vi "Run Tests Programmatically.vi"(4 "Verbose":bool=TRUE, 5 "Silent":bool, 6 "Interactive":bool=TRUE, 7 "Inspect Recursively":bool=TRUE, 9 "Report name":string, 10 "Output Folder":path, 11 "Source Folder":path) -> (0 "error out":errorcluster, 3 "Test Runner":refnum<class "Test Runner.lvclass">)   [LabVIEW 2013, in "Caraya.lvlib"]
uses:
  Caraya.lvlib
  classes/Test Runner/Test Runner.lvclass
  <vilib>/Utility/error.llb/DialogType.ctl
  classes/Test Runner/Test Runner.lvclass/Test Runner.ctl
  classes/Test Runner.Folder/Test Runner.Folder.lvclass
  <userlib>/_OpenG.lib/file/file.llb/File Exists - Scalar__ogtk.vi
  <userlib>/_OpenG.lib/file/file.llb/Valid Path - Traditional__ogtk.vi
  <userlib>/_OpenG.lib/array/array.llb/Delete Elements from 1D Array (Path)__ogtk.vi
  <userlib>/_OpenG.lib/file/file.llb/Strip Path - Arrays__ogtk.vi
  <userlib>/_OpenG.lib/file/file.llb/Strip Path Extension - 1D Array of Strings__ogtk.vi
  <userlib>/_OpenG.lib/file/file.llb/Strip Path Extension - String__ogtk.vi
  <userlib>/_OpenG.lib/file/file.llb/Convert File Extension (String)__ogtk.vi
  classes/Test Report.JUnit/Test Report.JUnit.lvclass
  classes/Test Report.Default/Test Report.Default.lvclass
panel:
  in  "report format":enum16{"Plain text", "JUnit (XML)"}(ring)=enum."JUnit (XML)"
  in  "Defined Tests":i32[](listbox)
  in  "Run Batch Test":bool
  # "CARAYA Batch Testing\n\nFill in the source folder where your tests are and choose the output result options."
  # "Output Configuration"
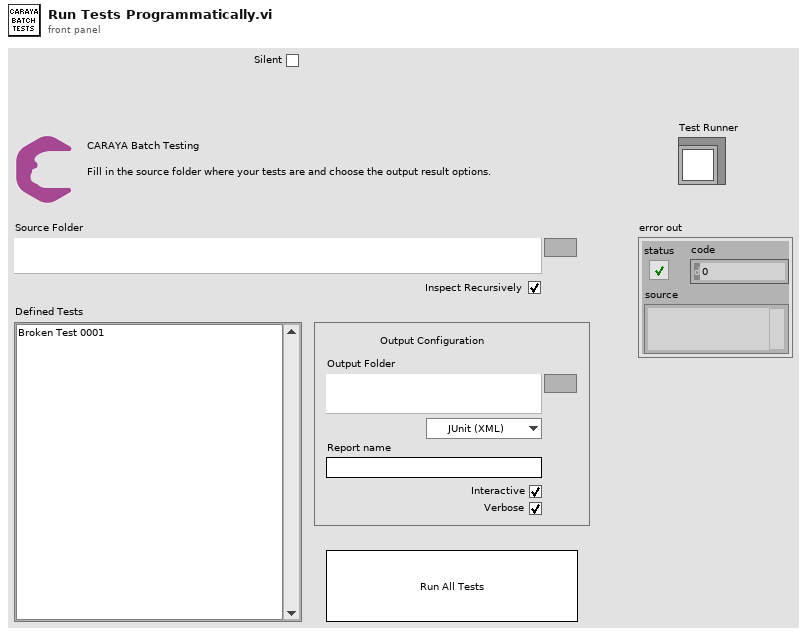
[diagram p1: front panel]
types:
  T1 = enum32{"invalid app kind", "Development System", "Run Time System", "Student Edition", "Embedded LabVIEW", "Evaluation", "Custom"}
  T2 = enum8{"Enabled", "Disabled", "Disabled and Grayed Out"}
  T3 = enum32{"Invalid", "Standard", "Closed", "Hidden", "Minimized", "Maximized"}
  T4 = cluster{"Core":cluster{"Current VI Reference":refnum<vi>, "Close Panel on Exit?":bool}, "Output Folder":path, "Report name":string, "Source Folder":path, "Interactive":bool, "Verbose":bool, "Menu Launch AppRef":refnum<vi>, "Silent":bool, "report format":enum16{"Plain text", "JUnit (XML)"}, "Test Runner":refnum<class "Test Runner.Folder.lvclass">}
  T5 = typedef "DialogType.ctl" = u16
  T6 = cluster{"Current VI Reference":refnum<vi>, "Close Panel on Exit?":bool}
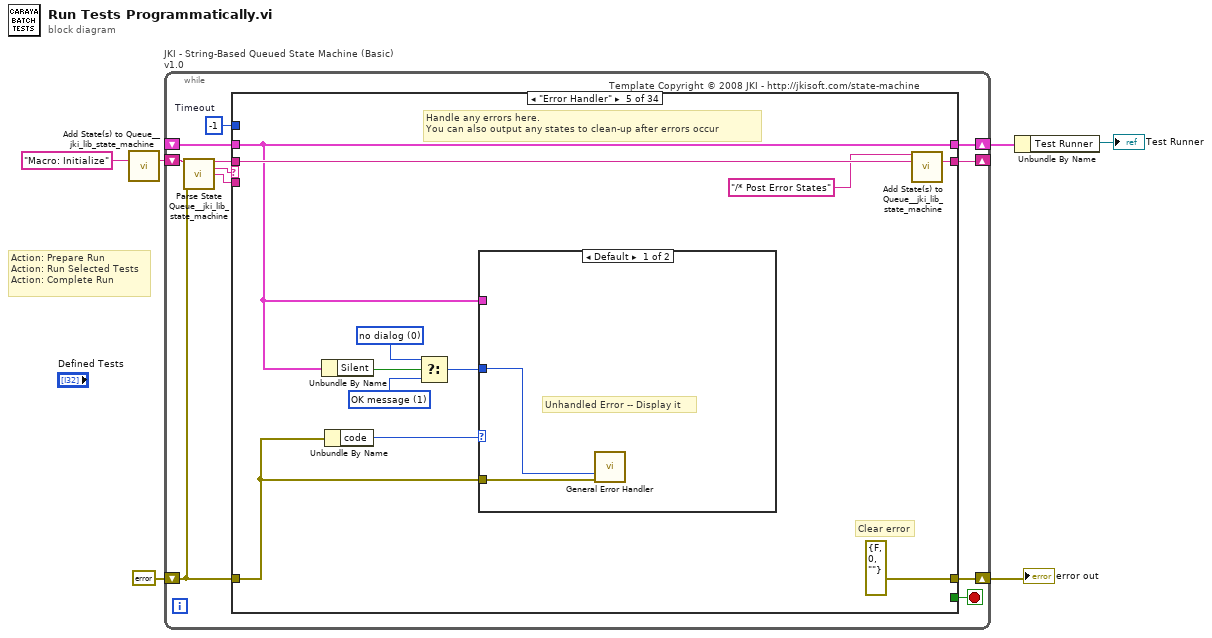
[diagram p0: block diagram]
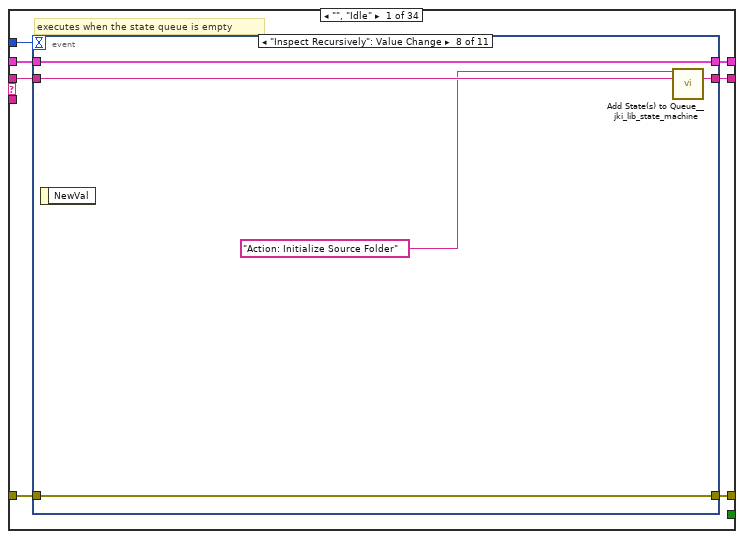
[diagram p2: hidden frame]
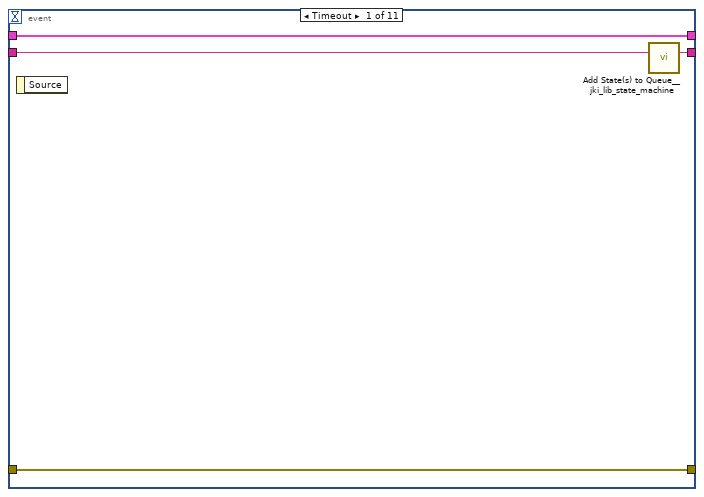
[diagram p3: hidden frame]
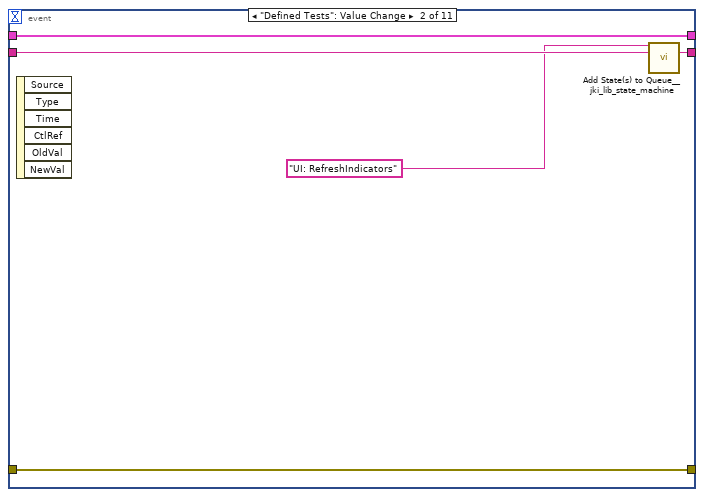
[diagram p4: hidden frame]
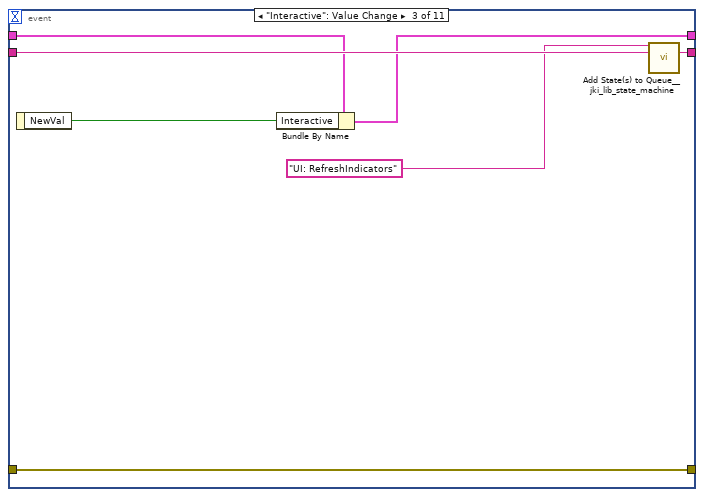
[diagram p5: hidden frame]
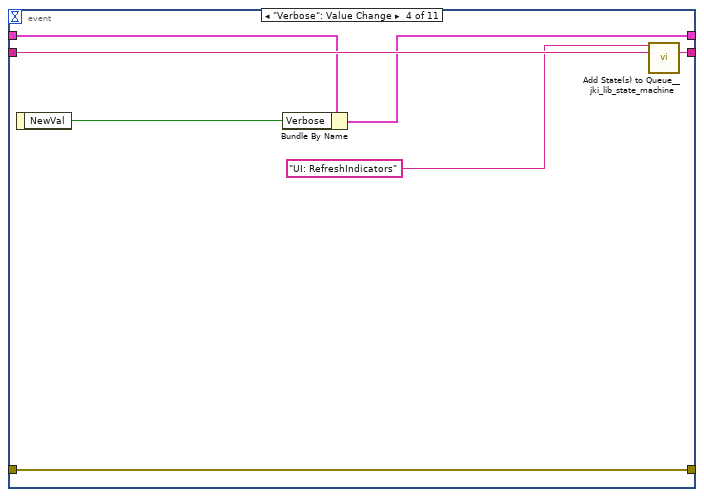
[diagram p6: hidden frame]
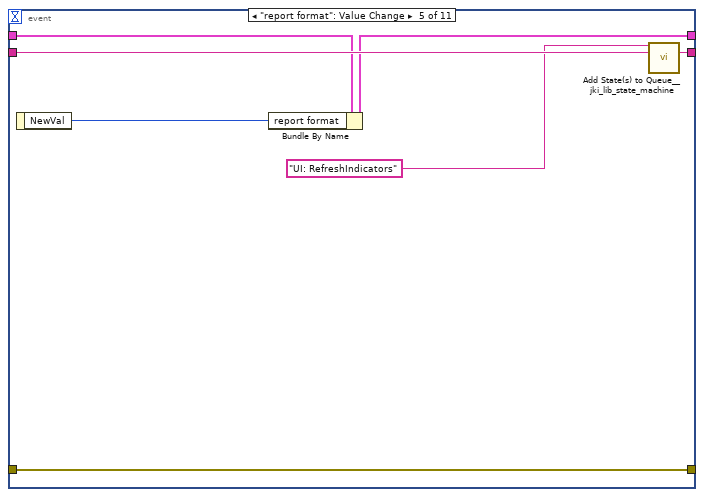
[diagram p7: hidden frame]
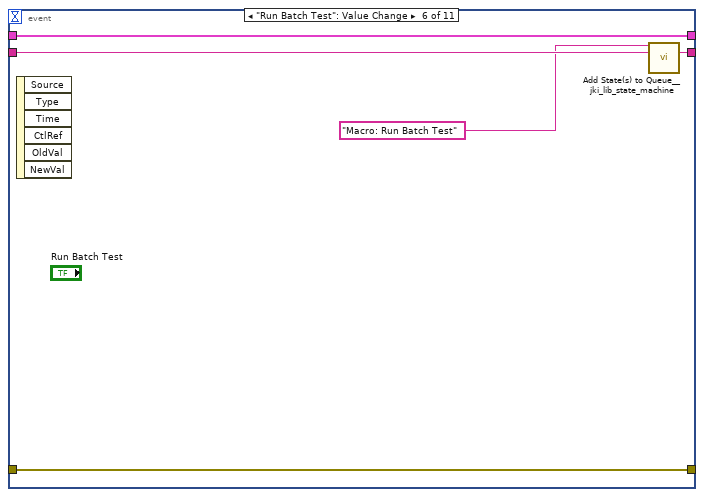
[diagram p8: hidden frame]
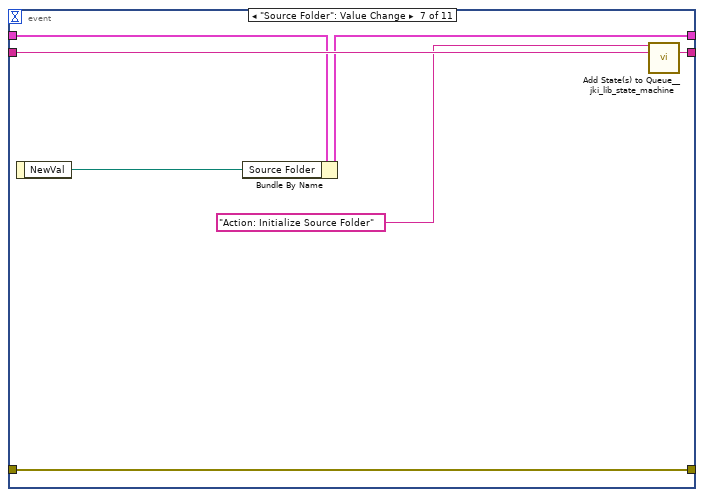
[diagram p9: hidden frame]
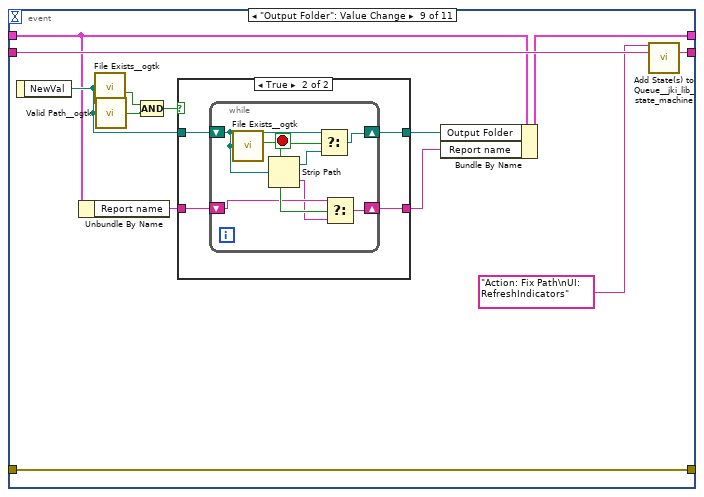
[diagram p10: hidden frame]
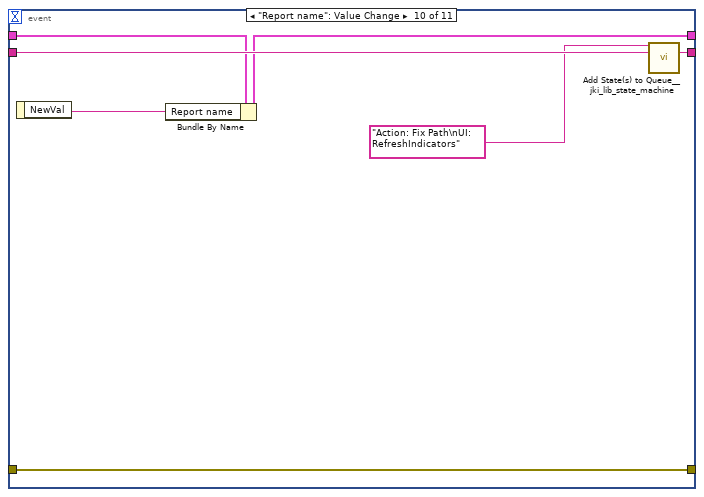
[diagram p12: hidden frame]
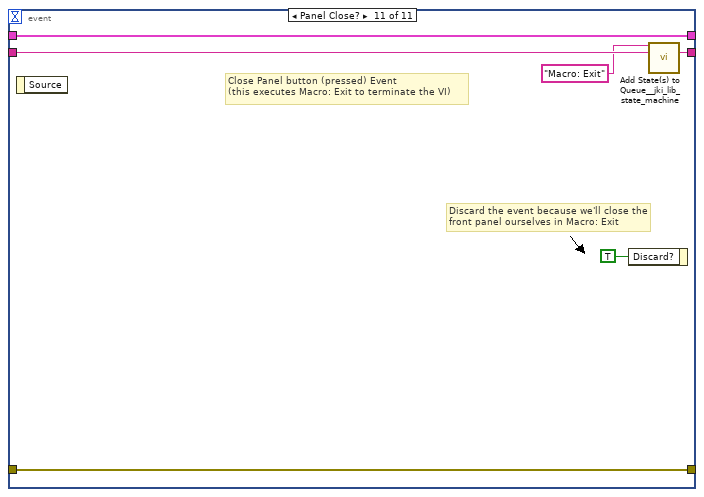
[diagram p13: hidden frame]
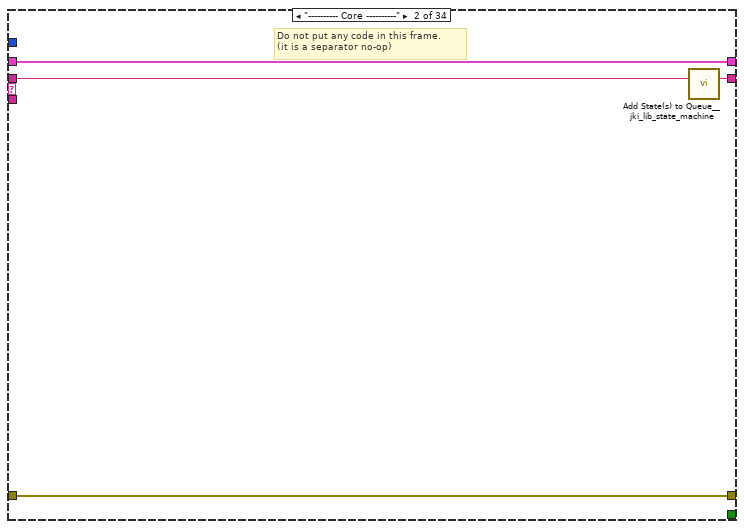
[diagram p14: hidden frame]
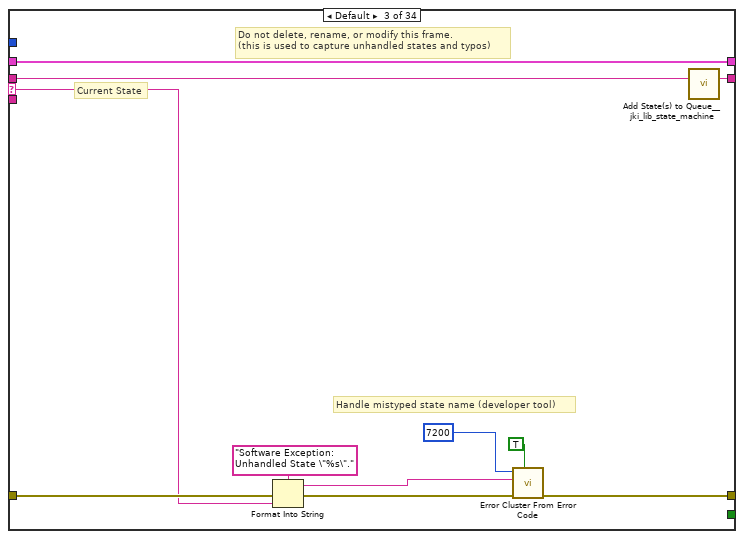
[diagram p15: hidden frame]
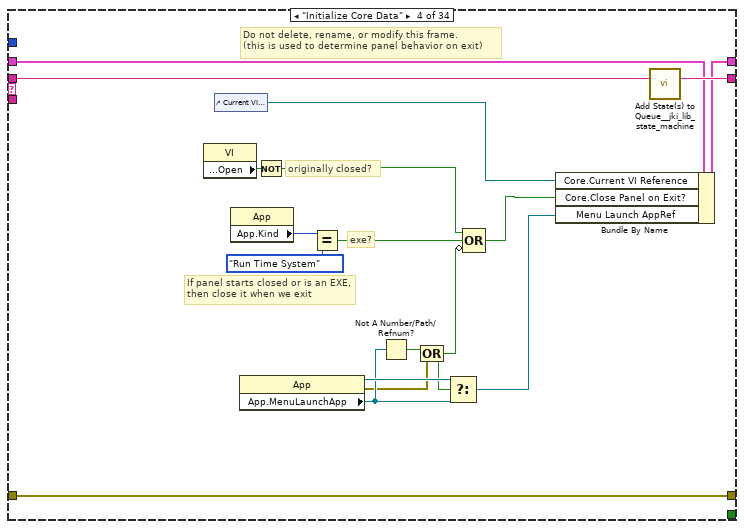
[diagram p16: hidden frame]
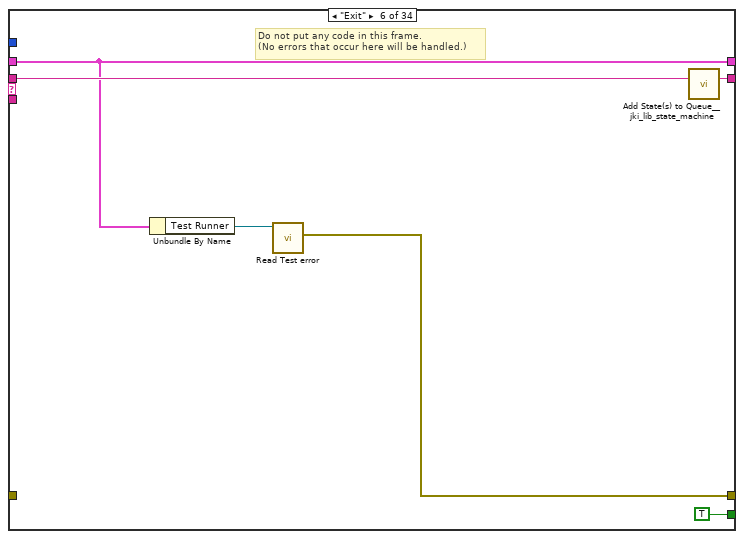
[diagram p18: hidden frame]
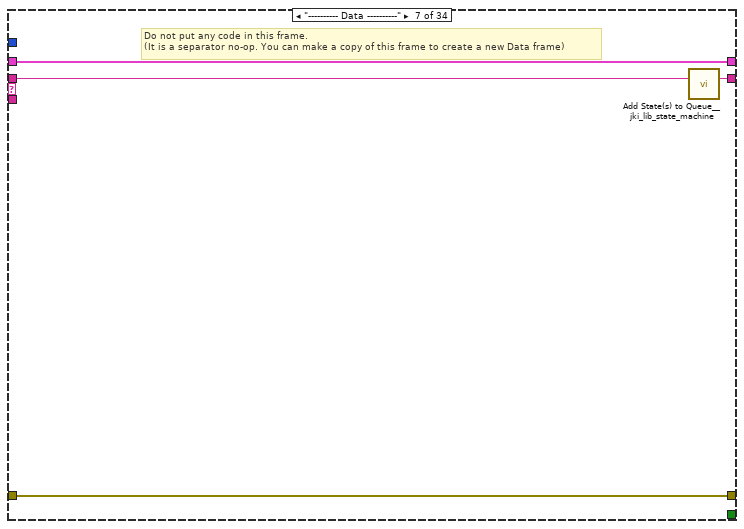
[diagram p19: hidden frame]
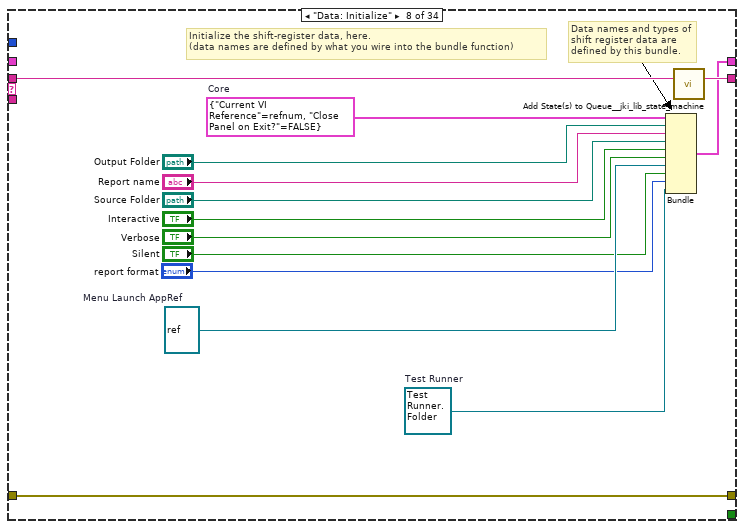
[diagram p20: hidden frame]
diagram:
  # "Action: Prepare Run\nAction: Run Selected Tests\nAction: Complete Run"
  n1 = call <vilib>:"Add State(s) to Queue__jki_lib_state_machine.vi"("State(s) in (\"\")"="Macro: Initialize") -> ("States Out"=w6:string)  [unwired: 14 in]
  n2 = while "JKI - String-Based Queued State Machine (Basic) v1.0" {
    shift-right: [w10] -> w2
    shift-left: _ -> [w9]
    shift-right: [w13] -> w4
    shift-left: errorcluster {"status"=FALSE, "code"=0, "source"=""} ("error IO") -> [w7]
    shift-right: [w12] -> _
    shift-left: w6 -> [w14]
    stop <- w11 stop-if-true
    w8 = -1  # Timeout
    # "Template Copyright © 2008 JKI - http://jkisoft.com/state-machine"
    n3 = call <vilib>:"Parse State Queue__jki_lib_state_machine.vi"("State Queue"=w14, "Error In (no error)"=w7) -> ("Remaining States"=w16:string, "Current State"=w17:string, "Arguments"=w15:string)  [unwired: 11 in]
    n4 = case shown="\"Error Handler\"" w17 {
      selector: w17 -> [_ _ w116 _ _ _ _ _ _ _ _ _ _ _ _ _ _ _ _ _ _ _ _ _ _ _ _ _ _ _ _ _ _ _]
      tunnel: w16 -> [w24 w114 w120 w143 w154 w162 w166 w180 w186 w190 w199 w234 w253 w264 w273 w285 w316 w321 w326 w331 w336 w341 w346 w352 w361 w366 w384 w418 w452 w467 w481 w488 w509 w529]
      tunnel: w15 -> [_ _ _ _ _ _ _ _ _ _ _ _ _ _ w268 w279 _ _ _ _ _ _ _ _ _ _ _ _ _ _ _ _ _ _]
      tunnel: w9 -> [w22 w111 w118 w135 w144 w159 w163 _ w181 w187 w195 w228 w251 w262 w271 w281 w313 w317 w323 w328 w333 w338 w343 w348 w358 w363 w381 w415 w450 w465 w478 w485 w497 w526]
      tunnel: [w21 w112 w122 w140 errorcluster {"status"=FALSE, "code"=0, "source"=""} ("error out") w157 w164 w177 w182 w188 w197 w232 w237 w257 w269 w282 w314 w319 w324 w329 w334 w339 w344 w350 w359 w364 w382 w416 w447 w462 w468 w486 w501 w527] -> w13
      tunnel: w7 -> [w20 w112 w121 w140 w149 _ w164 w177 w183 w188 w197 w232 w237 w258 w270 w283 w314 w319 w324 w329 w334 w339 w344 w350 w359 w364 w382 w416 w443 w460 w469 w486 w502 w527]
      tunnel: [w23 w113 w119 w142 w153 w161 w165 w179 w185 w189 w198 w233 w252 w263 w272 w284 w315 w320 w325 w330 w335 w340 w345 w351 w360 w365 w383 w417 w451 w466 w480 w487 w508 w528] -> w12
      tunnel: [_ _ _ _ _ TRUE _ _ _ _ _ _ _ _ _ _ _ _ _ _ _ _ _ _ _ _ _ _ _ _ _ _ _ _] -> w11
      tunnel: [w19 w111 w118 w141 w144 w159 w163 w178 w181 w187 w194 w227 w250 w262 w271 w281 w313 w317 w323 w328 w333 w338 w343 w348 w358 w363 w375 w414 w449 w464 w477 w485 w503 w526] -> w10
      tunnel: w8 -> [w18 _ _ _ _ _ _ _ _ _ _ _ _ _ _ _ _ _ _ _ _ _ _ _ _ _ _ _ _ _ _ _ _ _]
      frame "", "Idle" {
        # "executes when the state queue is empty"
        n5 = event shown="[7] \"Inspect Recursively\": Value Change" {
          selector: _ -> [_ _ _ _ _ _ _ _ _ _ _]
          dyn-events: _ -> [_ _ _ _ _ _ _ _ _ _ _]
          timeout: w18 -> [_ _ _ _ _ _ _ _ _ _ _]
          tunnel: w24 -> [w28 w33 w40 w47 w54 w59 w66 w71 w84 w104 w110]
          tunnel: [w27 w32 w39 w46 w53 w58 w65 w70 w83 w103 w109] -> w23
          tunnel: w22 -> [w25 w30 w35 w42 w49 w56 w61 w67 w74 w101 w107]
          tunnel: [w26 w31 w38 w45 w52 w57 w64 w69 w82 w102 w108] -> w21
          tunnel: w20 -> [w26 w31 w38 w45 w52 w57 w64 w69 w82 w102 w108]
          tunnel: [w25 w30 w34 w41 w48 w56 w63 w67 w81 w100 w107] -> w19
          event Timeout {
            n6 = event-data() -> ()  [unwired: 1 in, 1 out]
            n7 = call <vilib>:"Add State(s) to Queue__jki_lib_state_machine.vi"("State(s) in (\"\")"=w28) -> ("States Out"=w27:string)  [unwired: 14 in]
          }
          event "Defined Tests": Value Change {
            n8 = event-data() -> ()  [unwired: 1 in, 6 out]
            n9 = call <vilib>:"Add State(s) to Queue__jki_lib_state_machine.vi"("State(s) in Front (\"\")"="UI: RefreshIndicators", "State(s) in (\"\")"=w33) -> ("States Out"=w32:string)  [unwired: 13 in]
          }
          event "Interactive": Value Change {
            n10 = event-data() -> ("NewVal"=w36:bool)  [unwired: 1 in]
            n11 = Bundle By Name(cluster=w35, "Interactive"=w36) -> (w34:T4)
            n12 = call <vilib>:"Add State(s) to Queue__jki_lib_state_machine.vi"("State(s) in Front (\"\")"="UI: RefreshIndicators", "State(s) in (\"\")"=w40) -> ("States Out"=w39:string)  [unwired: 13 in]
          }
          event "Verbose": Value Change {
            n13 = event-data() -> ("NewVal"=w43:bool)  [unwired: 1 in]
            n14 = Bundle By Name(cluster=w42, "Verbose"=w43) -> (w41:T4)
            n15 = call <vilib>:"Add State(s) to Queue__jki_lib_state_machine.vi"("State(s) in Front (\"\")"="UI: RefreshIndicators", "State(s) in (\"\")"=w47) -> ("States Out"=w46:string)  [unwired: 13 in]
          }
          event "report format": Value Change {
            n16 = event-data() -> ("NewVal"=w50:enum16{"Plain text", "JUnit (XML)"})  [unwired: 1 in]
            n17 = Bundle By Name(cluster=w49, "report format"=w50) -> (w48:T4)
            n18 = call <vilib>:"Add State(s) to Queue__jki_lib_state_machine.vi"("State(s) in Front (\"\")"="UI: RefreshIndicators", "State(s) in (\"\")"=w54) -> ("States Out"=w53:string)  [unwired: 13 in]
          }
          event "Run Batch Test": Value Change {
            n19 = event-data() -> ()  [unwired: 1 in, 6 out]
            n20 = call <vilib>:"Add State(s) to Queue__jki_lib_state_machine.vi"("State(s) in Front (\"\")"="Macro: Run Batch Test", "State(s) in (\"\")"=w59) -> ("States Out"=w58:string)  [unwired: 13 in]
          }
          event "Source Folder": Value Change {
            n21 = event-data() -> ("NewVal"=w60:path)  [unwired: 1 in]
            n22 = Bundle By Name(cluster=w61, "Source Folder"=w60) -> (w63:T4)
            n23 = call <vilib>:"Add State(s) to Queue__jki_lib_state_machine.vi"("State(s) in Front (\"\")"="Action: Initialize Source Folder", "State(s) in (\"\")"=w66) -> ("States Out"=w65:string)  [unwired: 13 in]
          }
          event "Inspect Recursively": Value Change {
            n24 = event-data() -> ()  [unwired: 1 in, 1 out]
            n25 = call <vilib>:"Add State(s) to Queue__jki_lib_state_machine.vi"("State(s) in Front (\"\")"="Action: Initialize Source Folder", "State(s) in (\"\")"=w71) -> ("States Out"=w70:string)  [unwired: 13 in]
          }
          event "Output Folder": Value Change {
            n26 = event-data() -> ("NewVal"=w77:path)  [unwired: 1 in]
            n27 = Unbundle By Name(w74) -> ("Report name"=w73:string)
            n28 = call-poly <userlib>:"File Exists__ogtk.vi"("file path"=w77) -> ("exists"=w79:bool)  [unwired: 6 in, 1 out]
            n29 = call-poly <userlib>:"Valid Path__ogtk.vi"("path"=w77) -> ("valid"=w80:bool)
            n30 = Compound Arithmetic op=AND(w79, w80) -> (w78:bool)
            n31 = case shown="True" w78 {
              tunnel: w77 -> [w86 w90]
              tunnel: [w86 w89] -> w76
              tunnel: w73 -> [w85 w88]
              tunnel: [w85 w87] -> w72
              frame False {
              }
              frame True {
                n32 = while {
                  shift-right: [w97] -> w89
                  shift-left: w90 -> [w96]
                  shift-right: [w91] -> w87
                  shift-left: w88 -> [w93]
                  stop <- w94 stop-if-true
                  n33 = call-poly <userlib>:"File Exists__ogtk.vi"("file path"=w96) -> ("is directory"=w94:bool)  [unwired: 6 in, 1 out]
                  n34 = Strip Path(path=w96) -> (stripped path=w95:path, name=w92:string)
                  n35 = Select(t=w96, s=w94, f=w95) -> (s? t:f=w97:path)
                  n36 = Select(t=w93, s=w94, f=w92) -> (s? t:f=w91:string)
                }
              }
            }
            n37 = Bundle By Name(cluster=w74, "Output Folder"=w76, "Report name"=w72) -> (w81:T4)
            n38 = call <vilib>:"Add State(s) to Queue__jki_lib_state_machine.vi"("State(s) in Front (\"\")"="Action: Fix Path\nUI: RefreshIndicators", "State(s) in (\"\")"=w84) -> ("States Out"=w83:string)  [unwired: 13 in]
          }
          event "Report name": Value Change {
            n39 = event-data() -> ("NewVal"=w99:string)  [unwired: 1 in]
            n40 = Bundle By Name(cluster=w101, "Report name"=w99) -> (w100:T4)
            n41 = call <vilib>:"Add State(s) to Queue__jki_lib_state_machine.vi"("State(s) in Front (\"\")"="Action: Fix Path\nUI: RefreshIndicators", "State(s) in (\"\")"=w104) -> ("States Out"=w103:string)  [unwired: 13 in]
          }
          event Panel Close? {
            # "Discard the event because we'll close the front panel ourselves in Macro: Exit"
            # "Close Panel button (pressed) Event\n(this executes Macro: Exit to terminate the VI)"
            n42 = event-data() -> ()  [unwired: 1 in, 1 out]
            n43 = event-data("Discard?"=TRUE) -> ()  [unwired: 1 in, 1 out]
            n44 = call <vilib>:"Add State(s) to Queue__jki_lib_state_machine.vi"("State(s) in Front (\"\")"="Macro: Exit", "State(s) in (\"\")"=w110) -> ("States Out"=w109:string)  [unwired: 13 in]
          }
        }
      }
      frame "---------- Core ----------" {
        # "Do not put any code in this frame.\n(it is a separator no-op)"
        n45 = call <vilib>:"Add State(s) to Queue__jki_lib_state_machine.vi"("State(s) in (\"\")"=w114) -> ("States Out"=w113:string)  [unwired: 14 in]
      }
      frame Default {
        # "Current State"
        # "Do not delete, rename, or modify this frame.\n(this is used to capture unhandled states and typos)"
        # "Handle mistyped state name (developer tool)"
        n46 = Format Into String(format string="Software Exception: Unhandled State \"%s\"." ("message"), error in=w121, w116) -> (resulting string=w124:string, error out=w123:errorcluster)  [unwired: 1 in]
        n47 = call <vilib>:"Error Cluster From Error Code.vi"("show call chain? (False)"=TRUE, "error in (no error)"=w123, "error message (\"\")"=w124, "error code (0)"=7200) -> ("error out"=w122:errorcluster)  [unwired: 5 in]
        n48 = call <vilib>:"Add State(s) to Queue__jki_lib_state_machine.vi"("State(s) in (\"\")"=w120) -> ("States Out"=w119:string)  [unwired: 14 in]
      }
      frame "Initialize Core Data" {
        # "Do not delete, rename, or modify this frame.\n(this is used to determine panel behavior on exit)"
        # "originally closed?"
        # "exe?"
        # "If panel starts closed or is an EXE, then close it when we exit"
        n49 = property class="VI"() -> ("Front Panel.Open"=w139:bool)  [unwired: 2 in, 2 out]
        n50 = control-ref of="Current VI Reference"() -> (w136:refnum<vi>)
        n51 = property class="App"() -> ("App.Kind"=w138:T1)  [unwired: 2 in, 2 out]
        n52 = property class="App"() -> (reference out=w131:refnum<vi>, error out=w128:errorcluster, "App.MenuLaunchApp"=w130:refnum<vi>)  [unwired: 2 in]
        n53 = Not(x=w139) -> (.not. x?=w133:bool)
        n54 = Equal?(x=w138, y=T1."Run Time System" ("Application:Kind")) -> (x = y?=w132:bool)
        n55 = Not A Number/Path/Refnum?(number/path/refnum=w130) -> (NaN/Path/Refnum?=w127:bool)
        n56 = Compound Arithmetic op=OR(w127, w128) -> (w126:bool)
        n57 = Select(t=w131, s=w126, f=w130) -> (s? t:f=w129:refnum<vi>)
        n58 = Compound Arithmetic op=OR(w133, w132, invert w126) -> (w134:bool)
        n59 = Bundle By Name(cluster=w135, "Core.Current VI Reference"=w136, "Core.Close Panel on Exit?"=w134, "Menu Launch AppRef"=w129) -> (w141:T4)
        n60 = call <vilib>:"Add State(s) to Queue__jki_lib_state_machine.vi"("State(s) in (\"\")"=w143) -> ("States Out"=w142:string)  [unwired: 14 in]
      }
      frame "Error Handler" {
        w147 = T5 0 items=["no dialog", "OK message", "continue or stop message", "OK message + warnings", "continue/stop + warnings"] ("type of dialog (OK msg:1)")
        w146 = T5 1 items=["no dialog", "OK message", "continue or stop message", "OK message + warnings", "continue/stop + warnings"] ("type of dialog (OK msg:1)")
        # "Handle any errors here.\nYou can also output any states to clean-up after errors occur"
        # "Clear error"
        n61 = Unbundle By Name(w144) -> ("Silent"=w148:bool)
        n62 = Unbundle By Name(w149) -> ("code"=w150:i32)
        n63 = Select(t=w147, s=w148, f=w146) -> (s? t:f=w145:T5)
        n64 = case shown="Default" w150 {
          tunnel: w149 -> [w156 _]
          tunnel: w145 -> [w155 _]
          tunnel: w144 -> [_ _]
          frame Default {
            # "Unhandled Error -- Display it"
            n65 = call <vilib>:"General Error Handler.vi"("type of dialog (OK msg:1)"=w155, "error in (no error)"=w156) -> ()  [unwired: 9 in, 5 out]
          }
          frame 7000..7999 {
            # "Caraya Error Range"
          }
        }
        n66 = call <vilib>:"Add State(s) to Queue__jki_lib_state_machine.vi"("State(s) in Front (\"\")"="/* Post Error States", "State(s) in (\"\")"=w154) -> ("States Out"=w153:string)  [unwired: 13 in]
      }
      frame "Exit" {
        # "Do not put any code in this frame.\n(No errors that occur here will be handled.)"
        n67 = Unbundle By Name(w159) -> ("Test Runner"=w158:refnum<class "Test Runner.Folder.lvclass">)
        n68 = call "Read Test error.vi"("Test Runner in"=w158) -> ("Test error"=w157:errorcluster)  [unwired: 8 in, 2 out]
        n69 = call <vilib>:"Add State(s) to Queue__jki_lib_state_machine.vi"("State(s) in (\"\")"=w162) -> ("States Out"=w161:string)  [unwired: 14 in]
      }
      frame "---------- Data ----------" {
        # "Do not put any code in this frame.\n(It is a separator no-op. You can make a copy of this frame to create a new Data frame)"
        n70 = call <vilib>:"Add State(s) to Queue__jki_lib_state_machine.vi"("State(s) in (\"\")"=w166) -> ("States Out"=w165:string)  [unwired: 14 in]
      }
      frame "Data: Initialize" {
        w167 = refnum<class "Test Runner.Folder.lvclass"> refnum  # Test Runner
        w175 = refnum<vi> refnum  # Menu Launch AppRef
        w176 = T6 {"Current VI Reference"=refnum, "Close Panel on Exit?"=FALSE}  # Core
        # "Data names and types of shift register data are defined by this bundle."
        # "Initialize the shift-register data, here.\n(data names are defined by what you wire into the bundle function)"
        n71 = Bundle("Core"=w176, "Output Folder"="Output Folder", "Report name"="Report name", "Source Folder"="Source Folder", "Interactive"="Interactive", "Verbose"="Verbose", "Menu Launch AppRef"=w175, "Silent"="Silent", "report format"="report format", "Test Runner"=w167) -> (w178:T4)  [unwired: 1 in]
        n72 = call <vilib>:"Add State(s) to Queue__jki_lib_state_machine.vi"("State(s) in (\"\")"=w180) -> ("States Out"=w179:string)  [unwired: 14 in]
      }
      frame "Data: Cleanup" {
        # "Cleanup any data and references, here.\n(this is called automatically, by the Macro: Exit)"
        n73 = Unbundle By Name(w181) -> ("Core.Current VI Reference"=w184:refnum<vi>)
        n74 = Close Reference(reference=w184, error in (no error)=w183) -> (error out=w182:errorcluster)
        n75 = call <vilib>:"Add State(s) to Queue__jki_lib_state_machine.vi"("State(s) in (\"\")"=w186) -> ("States Out"=w185:string)  [unwired: 14 in]
      }
      frame "---------- UI ----------" {
        # "Do not put any code in this frame.\n(It is a separator no-op. You can make a copy of this frame to create a new UI frame)"
        n76 = call <vilib>:"Add State(s) to Queue__jki_lib_state_machine.vi"("State(s) in (\"\")"=w190) -> ("States Out"=w189:string)  [unwired: 14 in]
      }
      frame "UI: Initialize" {
        # "If Silent, do not set\ninteractive flag to True"
        # "Initialize the User Interface, here.\n(this is called automatically, by the Macro: Init)"
        n77 = Unbundle By Name(w195) -> ("Interactive"=w193:bool, "Silent"=w192:bool)
        n78 = Compound Arithmetic op=AND(w193, invert w192) -> (w191:bool)
        n79 = Bundle By Name(cluster=w195, "Interactive"=w191) -> (w194:T4)
        n80 = call <vilib>:"Add State(s) to Queue__jki_lib_state_machine.vi"("State(s) in Front (\"\")"="UI: Refresh Defined Tests\nAction: Fix Path\nUI: Initialize Path\nUI: RefreshIndicators" ("Text.Text"), "State(s) in (\"\")"=w199) -> ("States Out"=w198:string)  [unwired: 13 in]
      }
      frame "UI: RefreshIndicators" {
        n81 = Unbundle By Name(w228) -> ("Report name"=w210:string, "Output Folder"=w200:path, "Interactive"=w226:bool, "Source Folder"=w205:path, "report format"=w208:enum16{"Plain text", "JUnit (XML)"}, "Test Runner"=w218:refnum<class "Test Runner.Folder.lvclass">)
        n82 = property on="Defined Tests" class="LstBox (strict)"() -> ("Value"=w209:i32[])  [unwired: 2 in, 2 out]
        n83 = local write "Output Folder"(w200) -> ()
        n84 = local write "Report name"(w210) -> ()
        n85 = local write "Source Folder"(w205) -> ()
        n86 = local write "report format"(w208) -> ()
        n87 = call "Read Test VIs.vi"("Test Runner in"=w218) -> ("Test VIs"=w214:path[], "Test Runner out"=w215:refnum<class "Test Runner.Folder.lvclass">)  [unwired: 8 in, 1 out]
        n88 = call-poly <userlib>:"Valid Path__ogtk.vi"("path"=w200) -> ("valid"=w203:bool)
        n89 = call-poly <userlib>:"File Exists__ogtk.vi"("file path"=w200) -> ("is directory"=w202:bool, "exists"=w201:bool)  [unwired: 6 in]
        n90 = Empty Array?(array=w214) -> (empty?=w207:bool)
        n91 = Empty String/Path?(string/path=w200) -> (empty?=w204:bool)
        n92 = Empty Array?(array=w209) -> (empty?=w216:bool)
        n93 = call-poly <userlib>:"Delete Elements from Array__ogtk.vi"("indices"=w209, "array"=w214) -> ("array w/ subset deleted"=w213:path[])  [unwired: 8 in, 1 out]
        n94 = Array Size(array=w209) -> (size(s)=w221:i32)
        n95 = Select(t=path[] [], s=w207, f=w213) -> (s? t:f=w212:path[])
        n96 = Compound Arithmetic op=OR(w207, w204, invert w203, invert w202, invert w201) -> (w206:bool)
        n97 = Format Into String(format string="Run Selected Tests (%d)", w221) -> (resulting string=w219:string)  [unwired: 2 in, 1 out]
        n98 = call "Write Excluded Tests.vi"("Excluded Tests"=w212, "Test Runner in"=w215) -> ("Test Runner out"=w217:refnum<class "Test Runner.Folder.lvclass">)  [unwired: 8 in, 1 out]
        n99 = Select(t="Run All Tests", s=w216, f=w219) -> (s? t:f=w223:string)
        n100 = Bundle By Name(cluster=w228, "Interactive"=w226, "Test Runner"=w217) -> (w227:T4)
        n101 = Select(t="Run Tests", s=w206, f=w223) -> (s? t:f=w224:string)
        n102 = Select(t=T2."Disabled and Grayed Out" ("Disabled"), s=w206, f=T2."Enabled" ("Disabled")) -> (s? t:f=w229:T2)
        n103 = property on="Run Batch Test" class="Bool"("BoolText.Text"=w224) -> ()  [unwired: 2 in, 2 out]
        n104 = property on="Run Batch Test" class="Bool"("DisabledEnum"=w229) -> ()  [unwired: 2 in, 2 out]
        n105 = call <vilib>:"Add State(s) to Queue__jki_lib_state_machine.vi"("State(s) in (\"\")"=w234) -> ("States Out"=w233:string)  [unwired: 14 in]
      }
      frame "UI: Initialize Path" {
        n106 = Unbundle By Name(w251) -> ("Source Folder"=w244:path, "Output Folder"=w238:path)  [unwired: 1 out]
        n107 = call-poly <userlib>:"Valid Path__ogtk.vi"("path"=w238) -> ("valid"=w241:bool)
        n108 = call-poly <userlib>:"File Exists__ogtk.vi"("file path"=w238) -> ("is directory"=w239:bool, "exists"=w240:bool)  [unwired: 6 in]
        n109 = call-poly <userlib>:"Valid Path__ogtk.vi"("path"=w244) -> ("valid"=w247:bool)
        n110 = call-poly <userlib>:"File Exists__ogtk.vi"("file path"=w244) -> ("is directory"=w249:bool, "exists"=w248:bool)  [unwired: 6 in]
        n111 = Compound Arithmetic op=AND(w239, w240, w241) -> (w242:bool)
        n112 = Compound Arithmetic op=AND(w249, w248, w247) -> (w246:bool)
        n113 = Select(t=w238, s=w242, f=path "") -> (s? t:f=w235:path)
        n114 = Select(t=w244, s=w246, f=path "") -> (s? t:f=w243:path)
        n115 = Bundle By Name(cluster=w251, "Source Folder"=w243, "Output Folder"=w235) -> (w250:T4)
        n116 = call <vilib>:"Add State(s) to Queue__jki_lib_state_machine.vi"("State(s) in (\"\")"=w253) -> ("States Out"=w252:string)  [unwired: 14 in]
      }
      frame "UI: Refresh Defined Tests" {
        n117 = Unbundle By Name(w262) -> ("Test Runner"=w260:refnum<class "Test Runner.Folder.lvclass">)
        n118 = call "Read Test VIs.vi"("error in (no error)"=w258, "Test Runner in"=w260) -> ("error out"=w257:errorcluster, "Test VIs"=w259:path[])  [unwired: 7 in, 1 out]
        n119 = call-poly <userlib>:"Strip Path__ogtk.vi"("path"=w259) -> ("name"=w261:string[])  [unwired: 1 out]
        n120 = property on="Defined Tests" class="LstBox (strict)"() -> ("Item Names"=w255:string[])  [unwired: 2 in, 2 out]
        n121 = call-poly <userlib>:"Strip Path Extension__ogtk.vi"("paths"=w261) -> ("roots"=w256:string[])  [unwired: 1 out]
        n122 = Not Equal?(x=w256, y=w255) -> (x != y?=w254:bool)
        n123 = case shown="True" w254 {
          tunnel: w256 -> [_ w267]
          frame False {
          }
          frame True {
            n124 = property on="Defined Tests" class="LstBox (strict)"("Item Names"=w267, "Value"=i32[] [] ("Defined Tests"), "Top Row"=0) -> ()  [unwired: 2 in, 2 out]
          }
        }
        n125 = call <vilib>:"Add State(s) to Queue__jki_lib_state_machine.vi"("State(s) in (\"\")"=w264) -> ("States Out"=w263:string)  [unwired: 14 in]
      }
      frame "UI: Cursor Set" {
        # "Argument"
        # "Set and Unset Cursor Busy.\n(Usage: \"UI: Cursor Set >> Busy|Idle\")"
        n126 = case shown="\"Idle\", Default" w268 {
          tunnel: w270 -> [w275 w277]
          tunnel: [w274 w276] -> w269
          frame "Idle", Default {
            n127 = call <vilib>:"Unset Busy.vi"("error in (no error)"=w275) -> ("error out"=w274:errorcluster)  [unwired: 10 in]
          }
          frame "Busy" {
            n128 = call <vilib>:"Set Busy.vi"("error in (no error)"=w277) -> ("error out"=w276:errorcluster)  [unwired: 9 in, 1 out]
          }
        }
        n129 = call <vilib>:"Add State(s) to Queue__jki_lib_state_machine.vi"("State(s) in (\"\")"=w273) -> ("States Out"=w272:string)  [unwired: 14 in]
      }
      frame "UI: Front Panel State" {
        # "Argument"
        # "Set Front Panel Open or Closed\n(Usage: \"UI: Front Panel State >> Open|Close\")"
        n130 = Unbundle By Name(w281) -> ("Silent"=w278:bool, "Core.Current VI Reference"=w280:refnum<vi>)
        n131 = case shown="\"Open\", Default" w279 {
          tunnel: w283 -> [w287 w307]
          tunnel: [w289 w308] -> w282
          tunnel: w280 -> [w288 w305]
          tunnel: w278 -> [w286 _]
          frame "Open", Default {
            n132 = case shown="False" w286 {
              tunnel: [w295 w302] -> w289
              tunnel: w288 -> [w294 _]
              tunnel: w287 -> [w293 w302]
              frame False {
                n133 = property class="VI"(reference=w294, error in=w293) -> (reference out=w291:refnum<vi>, error out=w292:errorcluster, "Front Panel.Open"=w290:bool)
                n134 = case shown="True" w290 {
                  tunnel: [w298 w301] -> w295
                  tunnel: w292 -> [w297 w301]
                  tunnel: w291 -> [w296 _]
                  frame False {
                    n135 = invoke class="VI" method="FP.Open"(reference=w296, error in=w297, "Activate"=TRUE, "State"=T3."Standard") -> (error out=w298:errorcluster)  [unwired: 1 in, 4 out]
                  }
                  frame True {
                  }
                }
              }
              frame True {
                # "Running Silently. Do not open"
              }
            }
          }
          frame "Close" {
            n136 = property class="VI"(reference=w305, error in=w307) -> (reference out=w304:refnum<vi>, error out=w306:errorcluster, "Front Panel.Open"=w303:bool)
            n137 = case shown="True" w303 {
              tunnel: [w309 w312] -> w308
              tunnel: w306 -> [w309 w311]
              tunnel: w304 -> [_ w310]
              frame False {
              }
              frame True {
                n138 = invoke class="VI" method="FP.Close"(reference=w310, error in=w311) -> (error out=w312:errorcluster)  [unwired: 1 in, 2 out]
              }
            }
          }
        }
        n139 = call <vilib>:"Add State(s) to Queue__jki_lib_state_machine.vi"("State(s) in (\"\")"=w285) -> ("States Out"=w284:string)  [unwired: 14 in]
      }
      frame "---------- Macro ----------" {
        # "Do not put any code in this frame.\n(It is a separator no-op. You can make a copy of this frame to create a new Macro frame)"
        n140 = call <vilib>:"Add State(s) to Queue__jki_lib_state_machine.vi"("State(s) in (\"\")"=w316) -> ("States Out"=w315:string)  [unwired: 14 in]
      }
      frame "Macro: Initialize" {
        w318 = "Data: Initialize\nInitialize Core Data\nUI: Initialize\nUI: Front Panel State >> Open\nAction: Initialize Source Folder\nUI: RefreshIndicators\nMacro: Run Silently?\n"  # Data: Initialize Initialize Core Data UI: Initialize UI: Front Panel State >> Open Action: Initialize Source Folder UI: RefreshIndicators Macro: Run Silently?
        # "Initialization Macro\n(This is called once, when the VI starts)"
        n141 = call <vilib>:"Add State(s) to Queue__jki_lib_state_machine.vi"("State(s) in Front (\"\")"=w318, "State(s) in (\"\")"=w321) -> ("States Out"=w320:string)  [unwired: 13 in]
      }
      frame "Macro: ComputePath" {
        n142 = call <vilib>:"Add State(s) to Queue__jki_lib_state_machine.vi"("State(s) in Front (\"\")"="UI: RefreshIndicators", "State(s) in (\"\")"=w326) -> ("States Out"=w325:string)  [unwired: 13 in]
      }
      frame "Macro: AppendClassName" {
        n143 = call <vilib>:"Add State(s) to Queue__jki_lib_state_machine.vi"("State(s) in Front (\"\")"="UI: RefreshIndicators", "State(s) in (\"\")"=w331) -> ("States Out"=w330:string)  [unwired: 13 in]
      }
      frame "Macro: Find Defined Tests" {
        n144 = call <vilib>:"Add State(s) to Queue__jki_lib_state_machine.vi"("State(s) in Front (\"\")"="Action: Find All Defined Tests\nUI: Refresh Defined Tests\nUI: RefreshIndicators", "State(s) in (\"\")"=w336) -> ("States Out"=w335:string)  [unwired: 13 in]
      }
      frame "Macro: Clear Defined Tests" {
        n145 = call <vilib>:"Add State(s) to Queue__jki_lib_state_machine.vi"("State(s) in Front (\"\")"="Action: Reset\nUI: Refresh Defined Tests\nUI: RefreshIndicators", "State(s) in (\"\")"=w341) -> ("States Out"=w340:string)  [unwired: 13 in]
      }
      frame "Macro: Run Batch Test" {
        n146 = call <vilib>:"Add State(s) to Queue__jki_lib_state_machine.vi"("State(s) in Front (\"\")"="Action: Prepare Run\nAction: Run Selected Tests\nAction: Complete Run", "State(s) in (\"\")"=w346) -> ("States Out"=w345:string)  [unwired: 13 in]
      }
      frame "Macro: Run Silently?" {
        n147 = Unbundle By Name(w348) -> ("Silent"=w347:bool)
        n148 = case shown="True" w347 {
          tunnel: [_ "Macro: Run Batch Test\nMacro: Exit"] -> w349
          frame False {
          }
          frame True {
          }
        }
        n149 = call <vilib>:"Add State(s) to Queue__jki_lib_state_machine.vi"("State(s) in Front (\"\")"=w349, "State(s) in (\"\")"=w352) -> ("States Out"=w351:string)  [unwired: 13 in]
      }
      frame "Macro: Exit" {
        # "Exit Macro\n(This is called once, when the VI exits)"
        n150 = Unbundle By Name(w358) -> ("Core.Close Panel on Exit?"=w354:bool)
        n151 = case shown="True" w354 {
          tunnel: [_ "UI: Front Panel State >> Close"] -> w355
          frame False {
          }
          frame True {
          }
        }
        n152 = call <vilib>:"Add State(s) to Queue__jki_lib_state_machine.vi"("State(s) in Front (\"\")"=w355, "State(s) at Back (\"\")"="Data: Cleanup\nExit") -> ("States Out"=w356:string)  [unwired: 13 in]
        n153 = call <vilib>:"Add State(s) to Queue__jki_lib_state_machine.vi"("State(s) in Front (\"\")"=w356, "State(s) in (\"\")"=w361) -> ("States Out"=w360:string)  [unwired: 13 in]
      }
      frame "---------- Action ----------" {
        n154 = call <vilib>:"Add State(s) to Queue__jki_lib_state_machine.vi"("State(s) in (\"\")"=w366) -> ("States Out"=w365:string)  [unwired: 14 in]
      }
      frame "Action: Fix Path" {
        n155 = Unbundle By Name(w381) -> ("Output Folder"=w377:path, "Report name"=w374:string, "report format"=w372:enum16{"Plain text", "JUnit (XML)"})
        n156 = call-poly <userlib>:"File Exists__ogtk.vi"("file path"=w377) -> ("exists"=w379:bool)  [unwired: 6 in, 1 out]
        n157 = call-poly <userlib>:"Valid Path__ogtk.vi"("path"=w377) -> ("valid"=w380:bool)
        n158 = Compound Arithmetic op=AND(w379, w380) -> (w378:bool)
        n159 = case shown="True" w378 {
          tunnel: w377 -> [w392 w396]
          tunnel: [w392 w395] -> w376
          tunnel: w374 -> [w391 w394]
          tunnel: [w391 w393] -> w368
          frame False {
          }
          frame True {
            n160 = while {
              shift-right: [w403] -> w395
              shift-left: w396 -> [w402]
              shift-right: [w399] -> w393
              shift-left: w394 -> [w400]
              stop <- w398 stop-if-true
              n161 = call-poly <userlib>:"File Exists__ogtk.vi"("file path"=w402) -> ("is directory"=w398:bool)  [unwired: 6 in, 1 out]
              n162 = Strip Path(path=w402) -> (stripped path=w401:path, name=w397:string)
              n163 = Select(t=w400, s=w398, f=w397) -> (s? t:f=w399:string)
              n164 = Select(t=w402, s=w398, f=w401) -> (s? t:f=w403:path)
            }
          }
        }
        n165 = case shown="Default" w368 {
          selector: w368 -> [w404 _]
          tunnel: [w404 w405] -> w369
          frame Default {
          }
          frame "" {
            n166 = Get Date/Time In Seconds() -> (seconds since 1Jan1904=w407:timestamp)
            n167 = Format Into String(format string="%<%Y%m%d_%H%M%S>T", w407) -> (resulting string=w405:string)  [unwired: 2 in, 1 out]
          }
        }
        n168 = call-poly <userlib>:"Strip Path Extension__ogtk.vi"("path"=w368) -> ("root"=w370:string, "extension"=w373:string)
        n169 = case shown="Default" w373 {
          tunnel: w372 -> [_ _ w390]
          tunnel: [enum16{"Plain text", "XML"}."XML" ("report format") enum16{"Plain text", "XML"}."Plain text" ("report format") w390] -> w371
          tunnel: w370 -> [w385 w387 _]
          tunnel: w369 -> [_ _ w389]
          tunnel: [w385 w387 w389] -> w367
          frame "xml" {
          }
          frame "txt" {
          }
          frame Default {
          }
        }
        n170 = Bundle By Name(cluster=w381, "Output Folder"=w376, "Report name"=w367, "report format"=w371) -> (w375:T4)
        n171 = call <vilib>:"Add State(s) to Queue__jki_lib_state_machine.vi"("State(s) in (\"\")"=w384) -> ("States Out"=w383:string)  [unwired: 14 in]
      }
      frame "Action: Initialize Source Folder" {
        n172 = Unbundle By Name(w415) -> ("Source Folder"=w410:path)
        n173 = for {
          N: 2 -> [_]
          tunnel: [w420] -> w411
          shift-right: [w421] -> w409
          shift-left: w410 -> [w422]
          stop <- w420 stop-if-true
          n174 = call-poly <userlib>:"Valid Path__ogtk.vi"("path"=w422) -> ("valid"=w423:bool)
          n175 = call-poly <userlib>:"File Exists__ogtk.vi"("file path"=w422) -> ("exists"=w419:bool)  [unwired: 6 in, 1 out]
          n176 = Compound Arithmetic op=AND(w419, w423) -> (w420:bool)
          n177 = case shown="False" w420 {
            tunnel: w422 -> [_ w428]
            tunnel: [w426 w428] -> w421
            tunnel: [w425 _] -> _
            frame False {
              n178 = property class="App"() -> (error out=w424:errorcluster, "Project.ActiveProject"=w427:refnum<vi>)  [unwired: 2 in, 1 out]
              n179 = property class="Project"(reference=w427, error in=w424) -> (error out=w425:errorcluster, "Path"=w426:path)  [unwired: 1 out]
            }
            frame True {
            }
          }
        }
        n180 = case shown="True" w411 {
          tunnel: w409 -> [w430 w433]
          tunnel: [w430 w432] -> w413
          tunnel: ["Macro: Clear Defined Tests" "Macro: Find Defined Tests"] -> w412
          frame False {
          }
          frame True {
            n181 = while {
              shift-right: [w436] -> w432
              shift-left: w433 -> [w435]
              stop <- w437 stop-if-true
              n182 = call-poly <userlib>:"File Exists__ogtk.vi"("file path"=w435) -> ("is directory"=w437:bool)  [unwired: 6 in, 1 out]
              n183 = Strip Path(path=w435) -> (stripped path=w434:path)  [unwired: 1 out]
              n184 = Select(t=w435, s=w437, f=w434) -> (s? t:f=w436:path)
            }
          }
        }
        n185 = Bundle By Name(cluster=w415, "Source Folder"=w413) -> (w414:T4)
        n186 = call <vilib>:"Add State(s) to Queue__jki_lib_state_machine.vi"("State(s) in Front (\"\")"=w412, "State(s) in (\"\")"=w418) -> ("States Out"=w417:string)  [unwired: 13 in]
      }
      frame "Action: Find All Defined Tests" {
        n187 = Unbundle By Name(w450) -> ("Menu Launch AppRef"=w438:refnum<vi>, "Test Runner"=w446:refnum<class "Test Runner.Folder.lvclass">, "Source Folder"=w444:path)
        n188 = call "Setup TestRunner Folder.vi"("Inspect Recursively (T)"="Inspect Recursively", "error in (no error)"=w443, "Directory to search"=w444, "Test Runner.Folder"=w446) -> ("error out"=w440:errorcluster, "Test Runner.Folder out"=w442:refnum<class "Test Runner.Folder.lvclass">)  [unwired: 6 in]
        n189 = call "Write ApplicationRef.vi"("error in (no error)"=w440, "Application"=w438, "Test Runner in"=w442) -> ("error out"=w439:errorcluster, "Test Runner out"=w441:refnum<class "Test Runner.Folder.lvclass">)  [unwired: 7 in]
        n190 = call "Discover Tests.vi"("error in (no error)"=w439, "Test Runner in"=w441) -> ("error out"=w447:errorcluster, "Test Runner out"=w448:refnum<class "Test Runner.Folder.lvclass">)  [unwired: 8 in]
        n191 = Bundle By Name(cluster=w450, "Test Runner"=w448) -> (w449:T4)
        n192 = call <vilib>:"Add State(s) to Queue__jki_lib_state_machine.vi"("State(s) in (\"\")"=w452) -> ("States Out"=w451:string)  [unwired: 14 in]
      }
      frame "Action: Reset" {
        n193 = Unbundle By Name(w465) -> ("Menu Launch AppRef"=w453:refnum<vi>, "Test Runner"=w459:refnum<class "Test Runner.Folder.lvclass">, "Source Folder"=w461:path)
        n194 = local read "Inspect Recursively"() -> (w458:bool)
        n195 = call "Setup TestRunner Folder.vi"("Inspect Recursively (T)"=w458, "error in (no error)"=w460, "Directory to search"=w461, "Test Runner.Folder"=w459) -> ("error out"=w455:errorcluster, "Test Runner.Folder out"=w457:refnum<class "Test Runner.Folder.lvclass">)  [unwired: 6 in]
        n196 = call "Write ApplicationRef.vi"("error in (no error)"=w455, "Application"=w453, "Test Runner in"=w457) -> ("error out"=w454:errorcluster, "Test Runner out"=w456:refnum<class "Test Runner.Folder.lvclass">)  [unwired: 7 in]
        n197 = call "Discover Tests.vi"("error in (no error)"=w454, "Test Runner in"=w456) -> ("error out"=w462:errorcluster, "Test Runner out"=w463:refnum<class "Test Runner.Folder.lvclass">)  [unwired: 8 in]
        n198 = Bundle By Name(cluster=w465, "Test Runner"=w463) -> (w464:T4)
        n199 = call <vilib>:"Add State(s) to Queue__jki_lib_state_machine.vi"("State(s) in (\"\")"=w467) -> ("States Out"=w466:string)  [unwired: 14 in]
      }
      frame "Action: Run Selected Tests" {
        n200 = Unbundle By Name(w478) -> ("Test Runner"=w479:refnum<class "Test Runner.Folder.lvclass">)
        n201 = property on="Defined Tests" class="LstBox (strict)"() -> ("Value"=w473:i32[])  [unwired: 2 in, 2 out]
        n202 = call "Read Test VIs.vi"("Test Runner in"=w479) -> ("Test VIs"=w475:path[], "Test Runner out"=w476:refnum<class "Test Runner.Folder.lvclass">)  [unwired: 8 in, 1 out]
        n203 = Empty Array?(array=w473) -> (empty?=w472:bool)
        n204 = case shown="False" w472 {
          tunnel: w475 -> [w484 _]
          tunnel: [w483 _] -> w474
          tunnel: w473 -> [w482 _]
          frame False {
            n205 = call-poly <userlib>:"Delete Elements from Array__ogtk.vi"("indices"=w482, "array"=w484) -> ("array w/ subset deleted"=w483:path[])  [unwired: 8 in, 1 out]
          }
          frame True {
          }
        }
        n206 = call "Write Excluded Tests.vi"("Excluded Tests"=w474, "Test Runner in"=w476) -> ("Test Runner out"=w471:refnum<class "Test Runner.Folder.lvclass">)  [unwired: 8 in, 1 out]
        n207 = call "Run.vi"("error in (no error)"=w469, "Test Runner in"=w471) -> ("error out"=w468:errorcluster, "Test Runner out"=w470:refnum<class "Test Runner.Folder.lvclass">)  [unwired: 7 in, 1 out]
        n208 = Bundle By Name(cluster=w478, "Test Runner"=w470) -> (w477:T4)
        n209 = call <vilib>:"Add State(s) to Queue__jki_lib_state_machine.vi"("State(s) in (\"\")"=w481) -> ("States Out"=w480:string)  [unwired: 14 in]
      }
      frame "Action: Complete Run" {
        n210 = call <vilib>:"Add State(s) to Queue__jki_lib_state_machine.vi"("State(s) in (\"\")"=w488) -> ("States Out"=w487:string)  [unwired: 14 in]
      }
      frame "Action: Prepare Run" {
        n211 = Unbundle By Name(w497) -> ("Output Folder"=w504:path, "Report name"=w505:string, "report format"=w507:enum16{"Plain text", "JUnit (XML)"}, "Verbose"=w506:bool)  [unwired: 1 out]
        n212 = Unbundle By Name(w497) -> ("Menu Launch AppRef"=w489:refnum<vi>, "Interactive"=w495:bool, "Test Runner"=w498:refnum<class "Test Runner.Folder.lvclass">, "Source Folder"=w496:path)
        n213 = case shown="\"Plain text\", Default" w507 {
          tunnel: [w512 w519] -> w499
          tunnel: w506 -> [w510 w518]
          tunnel: w505 -> [w514 w525]
          tunnel: w504 -> [w515 w522]
          tunnel: [w511 w521] -> w500
          frame "Plain text", Default {
            n214 = call-poly <userlib>:"Convert File Extension__ogtk.vi"("new ending (none)"="txt", "file name"=w514) -> ("new filename"=w516:string)  [unwired: 1 out]
            n215 = Build Path(base path=w515, name or relative path=w516) -> (appended path=w513:path)
            n216 = call "Create DefaultReport.vi"("Verbose"=w510, "Report Path"=w513) -> ("error out"=w512:errorcluster, "Test Report.Default out"=w511:refnum<class "Test Report.Default.lvclass">)  [unwired: 8 in]
          }
          frame "JUnit (XML)" {
            n217 = call-poly <userlib>:"Convert File Extension__ogtk.vi"("new ending (none)"="xml", "file name"=w525) -> ("new filename"=w523:string)  [unwired: 1 out]
            n218 = Build Path(base path=w522, name or relative path=w523) -> (appended path=w520:path)
            n219 = call "Create JUnit Report.vi"("Verbose"=w518, "Report Path"=w520) -> ("error out"=w519:errorcluster, "Test Report.JUnit out"=w521:refnum<class "Test Report.JUnit.lvclass">)  [unwired: 8 in]
          }
        }
        n220 = local read "Inspect Recursively"() -> (w494:bool)
        n221 = call "Setup TestRunner Folder.vi"("Interactive (T)"=w495, "Inspect Recursively (T)"=w494, "error in (no error)"=w499, "Test Report"=w500, "Directory to search"=w496, "Test Runner.Folder"=w498) -> ("error out"=w491:errorcluster, "Test Runner.Folder out"=w493:refnum<class "Test Runner.Folder.lvclass">)  [unwired: 4 in]
        n222 = call "Write ApplicationRef.vi"("error in (no error)"=w491, "Application"=w489, "Test Runner in"=w493) -> ("error out"=w490:errorcluster, "Test Runner out"=w492:refnum<class "Test Runner.Folder.lvclass">)  [unwired: 7 in]
        n223 = Bundle By Name(cluster=w497, "Test Runner"=w492) -> (w503:T4)
        n224 = Merge Errors(w502, w490) -> (w501:errorcluster)
        n225 = call <vilib>:"Add State(s) to Queue__jki_lib_state_machine.vi"("State(s) in (\"\")"=w509) -> ("States Out"=w508:string)  [unwired: 14 in]
      }
      frame "---------- Template ----------" {
        n226 = call <vilib>:"Add State(s) to Queue__jki_lib_state_machine.vi"("State(s) in (\"\")"=w529) -> ("States Out"=w528:string)  [unwired: 14 in]
      }
    }
  }
  "error out" <- w4
  n227 = Unbundle By Name(w2) -> ("Test Runner"=→"Test Runner":refnum<class "Test Runner.Folder.lvclass">)
